vi "getPeaks.vi"(8 "error in (no error)":errorcluster, 9 "useWarmThre":bool, 10 "phase":T1, 11 "reference in":refnum<class "subject.lvclass">) -> (0 "error out":errorcluster, 3 "reference out":refnum<class "subject.lvclass">)   [LabVIEW 2015, in "subject.lvclass"]
uses:
  subject.lvclass
  phase.ctl
  <vilib>/measure/mamon.llb/Waveform Peak Detection for 1 Chan.vi
  <vilib>/measure/NI_MAPro.lvlib
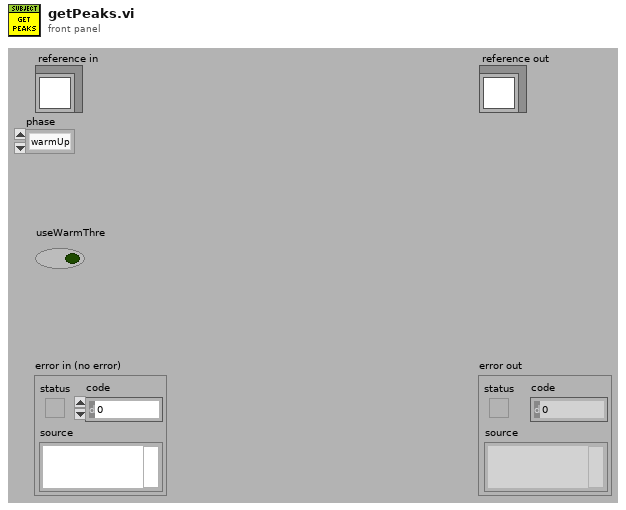
[diagram p1: front panel]
types:
  T1 = typedef "subject.lvclass/phase.ctl" = enum16{"warmUp", "Exercise"}
  T2 = cluster{"peaksAmplitude":dbl[], "iPeaksLocation":dbl[], "valesAmplitude":dbl[], "iValesLocation":dbl[], "threshold":dbl, "warmup_offset":i32, "exer_offset":i32, "#_peaks":i32}
  T3 = typedef "subject.lvclass/ObjectAttributesRef.ctl" = refnum<data-value>
  T4 = typedef "subject.lvclass/ObjectAttributes.ctl" = cluster{"MyAttribute":dbl, "data":cluster{"Ve_warm":dbl[], "time_warm":dbl[], "name":string, "phase":dbl[], "VCO2":dbl[], "VO2":dbl[], "PetCO2":dbl[], "RQ":dbl[], "HR":dbl[], "Ve_warm_inter":dbl[], "time_warm_inter":dbl[], "Ve_exer":dbl[], "time_exer":dbl[], "Ve_exer_inter":dbl[], "time_exer_inter":dbl[], "Ve":dbl[], "time":dbl[]}, "results_5l":cluster{"EOV":bool, "osci_amplitude":dbl[], "osci_width":dbl[], "peak_location":dbl[]}, "results_15percent":cluster{"EOV":bool, "osci_amplitude":dbl[], "osci_width":dbl[], "peak_location":dbl[]}, "supportData":cluster{"peaksAmplitude":dbl[], "iPeaksLocation":dbl[], "valesAmplitude":dbl[], "iValesLocation":dbl[], "threshold":dbl, "width_warm":i32, "meanAmpl_warm":i32, "#_peaks":i32}}
  T5 = cluster{"Ve_warm":dbl[], "time_warm":dbl[], "name":string, "phase":dbl[], "VCO2":dbl[], "VO2":dbl[], "PetCO2":dbl[], "RQ":dbl[], "HR":dbl[], "Ve_warm_inter":dbl[], "time_warm_inter":dbl[], "Ve_exer":dbl[], "time_exer":dbl[], "Ve_exer_inter":dbl[], "time_exer_inter":dbl[], "Ve":dbl[], "time":dbl[]}
  T6 = cluster{"peaksAmplitude":dbl[], "iPeaksLocation":dbl[], "valesAmplitude":dbl[], "iValesLocation":dbl[], "threshold":dbl, "width_warm":i32, "meanAmpl_warm":i32, "#_peaks":i32}
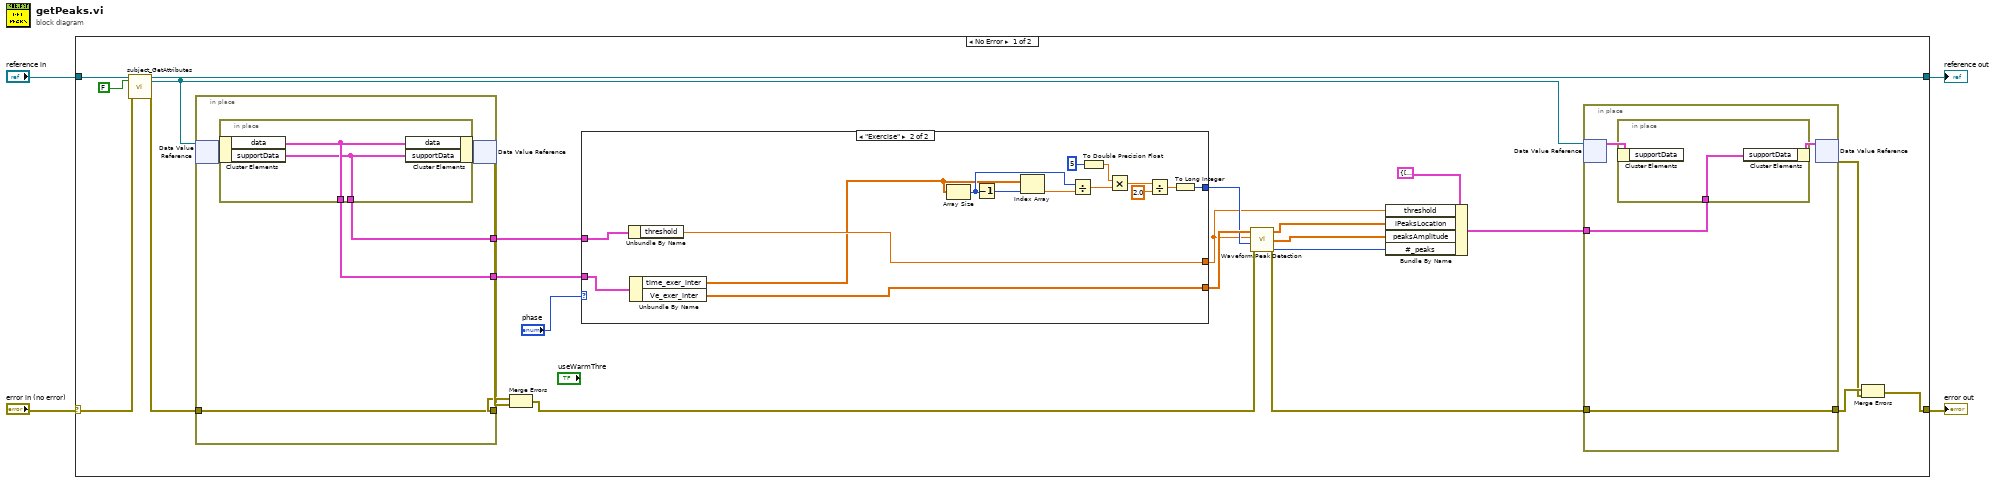
[diagram p0: block diagram]
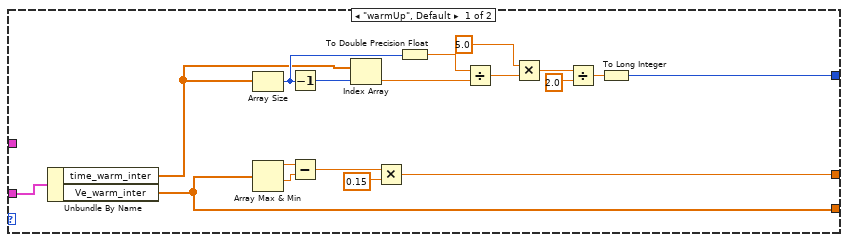
[diagram p2: hidden frame]
diagram:
  n1 = case shown="No Error" "error in (no error)" {
    selector: "error in (no error)" -> [w24 w75]
    tunnel: [w13 w75] -> w3
    tunnel: [w22 w74] -> w1
    tunnel: "reference in" -> [w26 w74]
    frame No Error {
      n2 = call "subject_GetAttributes.vi"("reference in"=w26, "return data? (T)"=FALSE, "error in (no error)"=w24) -> ("reference out"=w22:refnum<class "subject.lvclass">, "attributes ref"=w8:T3, "error out"=w23:errorcluster)  [unwired: 13 in, 1 out]
      n3 = in-place {
        in-place-border: w23 -> [w69]
        in-place-border: [w69] -> w27
        in-place-border: [w68] -> w20
        in-place-border: [w67] -> w7
        n4 = in-place-dvr #1(w8) -> (w70:T4)  [unwired: 1 out]
        n5 = in-place {
          in-place-border: [w73] -> w68
          in-place-border: [w72] -> w67
          n6 = in-place-cluster #2(w70) -> ("data"=w73:T5, "supportData"=w72:T6)
          n7 = in-place-cluster #2("data"=w73, "supportData"=w72) -> (w71:T4)
        }
        n8 = in-place-dvr #1(w71) -> (w28:errorcluster)  [unwired: 1 out]
      }
      n9 = Merge Errors(w27, w28) -> (w17:errorcluster)
      n10 = case shown="\"Exercise\"" "phase" {
        tunnel: w20 -> [w51 w66]
        tunnel: [w46 w64] -> w12
        tunnel: [w38 w54] -> w18
        tunnel: [w37 w53] -> w19
        tunnel: w7 -> [_ w65]
        frame "warmUp", Default {
          n11 = Unbundle By Name(w51) -> ("time_warm_inter"=w36:dbl[], "Ve_warm_inter"=w37:dbl[])
          n12 = Array Size(array=w36) -> (size(s)=w44:i32)
          n13 = Array Max & Min(array=w37) -> (max value=w50:dbl, min value=w49:dbl)  [unwired: 2 out]
          n14 = Decrement(x=w44) -> (x-1=w45:i32)
          n15 = Subtract(x=w50, y=w49) -> (x-y=w48:dbl)
          n16 = Index Array(array=w36, index=w45) -> (element=w43:dbl)
          n17 = Multiply(x=w48, y=0.15) -> (x*y=w46:dbl)
          n18 = To Double Precision Float(number=w44) -> (double precision float=w35:dbl)
          n19 = Divide(x=w35, y=w43) -> (x/y=w39:dbl)
          n20 = Multiply(x=5.0 ("Width (s):"), y=w39) -> (x*y=w42:dbl)
          n21 = Divide(x=w42, y=2.0) -> (x/y=w40:dbl)
          n22 = To Long Integer(number=w40) -> (32bit integer=w38:i32)
        }
        frame "Exercise" {
          n23 = Unbundle By Name(w65) -> ("threshold"=w64:dbl)
          n24 = Unbundle By Name(w66) -> ("time_exer_inter"=w52:dbl[], "Ve_exer_inter"=w53:dbl[])
          n25 = Array Size(array=w52) -> (size(s)=w62:i32)
          n26 = Decrement(x=w62) -> (x-1=w63:i32)
          n27 = Index Array(array=w52, index=w63) -> (element=w61:dbl)
          n28 = Divide(x=w62, y=w61) -> (x/y=w55:dbl)
          n29 = To Double Precision Float(number=5 ("Width (s):")) -> (double precision float=w60:dbl)
          n30 = Multiply(x=w60, y=w55) -> (x*y=w59:dbl)
          n31 = Divide(x=w59, y=2.0) -> (x/y=w57:dbl)
          n32 = To Long Integer(number=w57) -> (32bit integer=w54:i32)
        }
      }
      n33 = call-poly <vilib>:"Waveform Peak Detection.vi"("error in"=w17, "width"=w18, "threshold"=w12, "Signal In"=w19) -> ("error out"=w16:errorcluster, "Amplitudes"=w10:dbl[], "Locations"=w11:dbl[], "# found"=w5:i32)  [unwired: 3 in, 1 out]
      n34 = Bundle By Name(cluster=T2 {"peaksAmplitude"=[], "iPeaksLocation"=[], "valesAmplitude"=[], "iValesLocation"=[], "threshold"=0.0, "warmup_offset"=0, "exer_offset"=0, "#_peaks"=0} ("supportData"), "threshold"=w12, "iPeaksLocation"=w11, "peaksAmplitude"=w10, "#_peaks"=w5) -> (w9:T2)
      n35 = in-place {
        in-place-border: w16 -> [w30]
        in-place-border: [w30] -> w15
        in-place-border: w9 -> [w29]
        n36 = in-place-dvr #3(w8) -> (w31:T4)  [unwired: 1 out]
        n37 = in-place {
          in-place-border: w29 -> [w33]
          n38 = in-place-cluster #4(w31) -> ()  [unwired: 1 out]
          n39 = in-place-cluster #4("supportData"=w33) -> (w32:T4)
        }
        n40 = in-place-dvr #3(w32) -> (w14:errorcluster)  [unwired: 1 out]
      }
      n41 = Merge Errors(w15, w14) -> (w13:errorcluster)
    }
    frame Error {
    }
  }
  "error out" <- w3
  "reference out" <- w1
